vi "Log_Calib_Points.vi"(3 "Instrument type":T1=enum."Cross wire velocity", 4 "Root name":string, 5 "Calib file":path=path "/iMac_3 HD/Users/Hong(6%)/calib/XW Ch 1 7_10_02_6") -> ()   [LabVIEW 2010]
uses:
  Controls/Cal_Inst_type.ctl
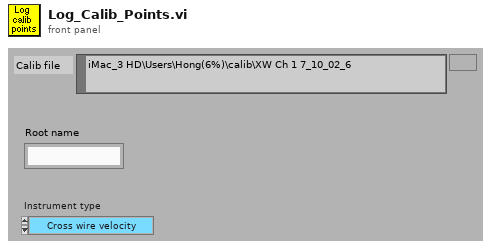
[diagram p1: front panel]
types:
  T1 = typedef "Cal_Inst_type.ctl" = enum16{"Propeller anemometer", "Pressure Transducer", "Hot wire", "Cross wire velocity", "Cross wire angle", "Generic Linear", "Generic Polynomial", "Generic BackPoly", "Fast FID", "Thermocouple", "Cold wire", "Pulsed Wire"}
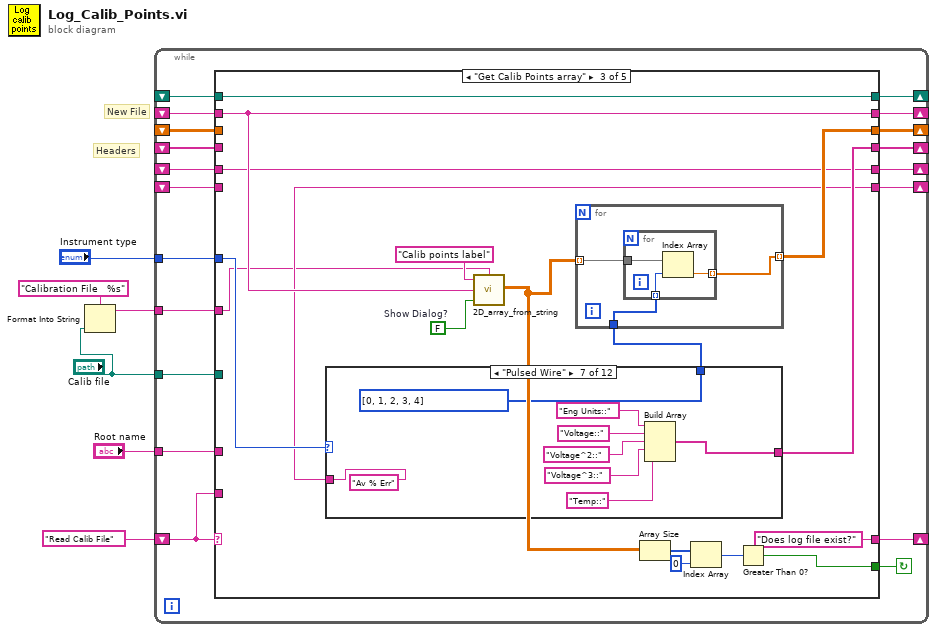
[diagram p0: block diagram]
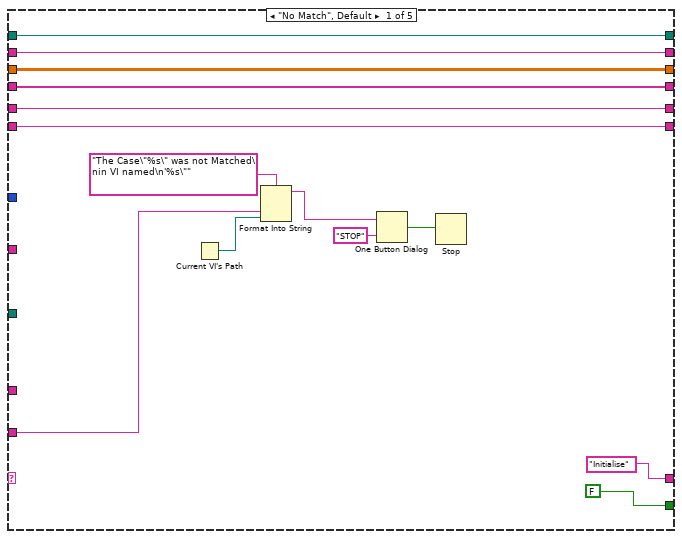
[diagram p2: hidden frame]
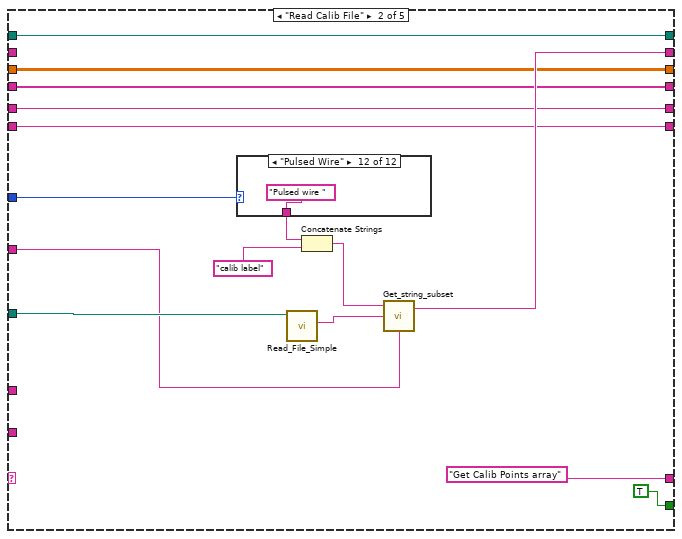
[diagram p3: hidden frame]
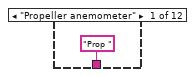
[diagram p4: hidden frame]
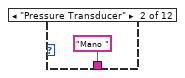
[diagram p5: hidden frame]
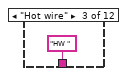
[diagram p6: hidden frame]
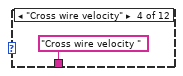
[diagram p7: hidden frame]
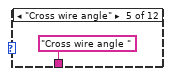
[diagram p8: hidden frame]
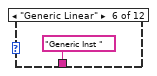
[diagram p9: hidden frame]
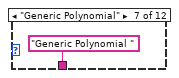
[diagram p10: hidden frame]
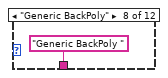
[diagram p11: hidden frame]
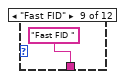
[diagram p12: hidden frame]
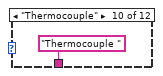
[diagram p13: hidden frame]
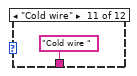
[diagram p14: hidden frame]
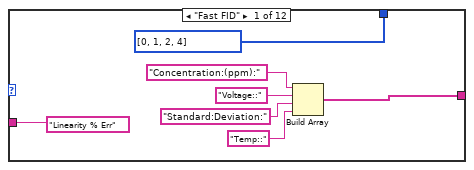
[diagram p15: hidden frame]
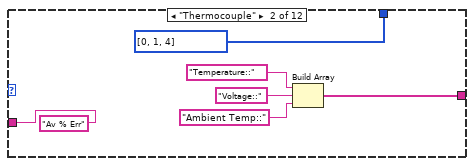
[diagram p16: hidden frame]
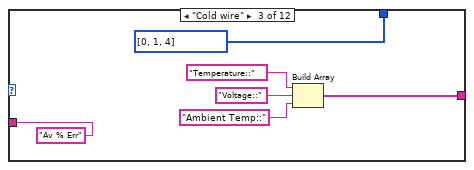
[diagram p17: hidden frame]
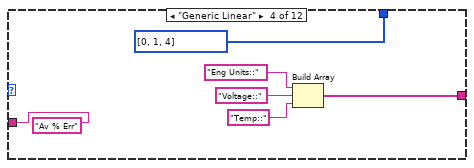
[diagram p18: hidden frame]
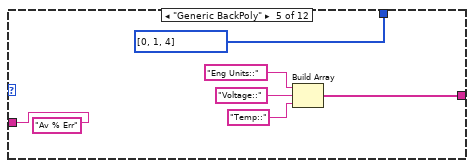
[diagram p19: hidden frame]
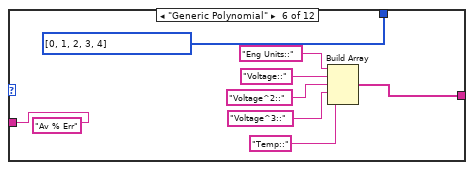
[diagram p20: hidden frame]
diagram:
  # "New File"
  # "Headers"
  n1 = Format Into String(format string="Calibration File   %s", "Calib file") -> (resulting string=w1:string)  [unwired: 2 in, 1 out]
  n2 = while {
    tunnel: "Calib file" -> [w15]
    shift-left: _ -> [w16]
    shift-right: [w17] -> _
    shift-left: _ -> [w18]
    shift-right: [w20] -> _
    tunnel: "Instrument type" -> [w22]
    shift-left: _ -> [w19]
    shift-right: [w21] -> _
    shift-left: "Read Calib File" -> [w23]
    shift-right: [w24] -> _
    tunnel: "Root name" -> [w14]
    shift-right: [w13] -> _
    shift-left: _ -> [w12]
    shift-right: [w11] -> _
    shift-left: _ -> [w10]
    shift-right: [w9] -> _
    shift-left: _ -> [w8]
    tunnel: w1 -> [w7]
    stop <- w25 continue-if-true
    n3 = case shown="\"Get Calib Points array\"" w23 {
      tunnel: [FALSE TRUE w77 TRUE FALSE] -> w25
      tunnel: ["Initialise" "Get Calib Points array" "Does log file exist?" "Append to log file" "End"] -> w24
      tunnel: w23 -> [w34 _ _ _ _]
      tunnel: w22 -> [_ w50 w81 _ _]
      tunnel: [w31 w49 w76 w176 w207] -> w21
      tunnel: [w30 w44 w70 w179 w220] -> w20
      tunnel: w19 -> [w31 _ w76 w176 w207]
      tunnel: w18 -> [w30 w44 _ w179 w220]
      tunnel: [w29 w48 w73 w180 w217] -> w17
      tunnel: w16 -> [w29 w48 _ w180 w217]
      tunnel: w15 -> [_ w41 _ _ w216]
      tunnel: w14 -> [_ _ _ w172 _]
      tunnel: [w28 w45 w71 w170 w199] -> w13
      tunnel: w12 -> [w28 w45 w71 _ w199]
      tunnel: [w27 w43 w69 w177 w214] -> w11
      tunnel: w10 -> [w27 w43 w69 _ w214]
      tunnel: [w26 w42 w68 w175 w200] -> w9
      tunnel: w8 -> [w26 w42 _ w175 w200]
      tunnel: w7 -> [_ w40 w67 _ _]
      frame "No Match", Default {
        n4 = Current VI's Path() -> (path=w33:path)
        n5 = Format Into String(format string="The Case\"%s\" was not Matched\nin VI named\n'%s\"" ("Format String"), w34, w33) -> (resulting string=w37:string)  [unwired: 2 in, 1 out]
        n6 = One Button Dialog(message=w37, button name ("OK")="STOP") -> (true=w35:bool)
        n7 = Stop(stop? (T)=w35) -> ()
      }
      frame "Read Calib File" {
        n8 = case shown="\"Pulsed Wire\"" w50 {
          tunnel: ["Prop " "Mano " "HW " "Cross wire velocity " "Cross wire angle " "Generic Inst " "Generic Polynomial " "Generic BackPoly " "Fast FID " "Thermocouple " "Cold wire " "Pulsed wire "] -> w51
          frame "Propeller anemometer" {
          }
          frame "Pressure Transducer" {
          }
          frame "Hot wire" {
          }
          frame "Cross wire velocity" {
          }
          frame "Cross wire angle" {
          }
          frame "Generic Linear" {
          }
          frame "Generic Polynomial" {
          }
          frame "Generic BackPoly" {
          }
          frame "Fast FID" {
          }
          frame "Thermocouple" {
          }
          frame "Cold wire" {
          }
          frame "Pulsed Wire" {
          }
        }
        n9 = call "Read_File_Simple.vi"("Filename"=w41) -> ("string"=w53:string)  [unwired: 2 in, 7 out]
        n10 = Concatenate Strings(w51, "calib label") -> (w47:string)
        n11 = call "Get_string_subset.vi"("String Name"=w40, "String to split"=w53, "File Label"=w47) -> ("Output string"=w49:string)  [unwired: 1 in, 1 out]
      }
      frame "Get Calib Points array" {
        w83 = FALSE  # Show Dialog?
        n12 = case shown="\"Pulsed Wire\"" w81 {
          tunnel: [i32[] [0, 1, 2, 4] i32[] [0, 1, 4] i32[] [0, 1, 4] i32[] [0, 1, 4] i32[] [0, 1, 4] i32[] [0, 1, 2, 3, 4] i32[] [0, 1, 2, 3, 4] i32[] [0, 1, 2, 3, 4] i32[] [0, 1, 2, 4] i32[] [0, 1, 4] i32[] [0, 1, 4] i32[] [0, 1, 4]] -> w75
          tunnel: [w93 w98 w104 w110 w116 w125 w133 w141 w148 w154 w160 w166] -> w70
          tunnel: ["Linearity % Err" "Av % Err" "Av % Err" "Av % Err" "Av % Err" "Av % Err" "Av % Err" "Av % Err" "Av % Err" "Av % Err" "Av % Err" "Av % Err"] -> w68
          frame "Fast FID" {
            n13 = Build Array("Concentration:(ppm):" ("Substring"), "Voltage::" ("Substring"), "Standard:Deviation:" ("Substring"), "Temp::" ("Substring")) -> (w93:string[])
          }
          frame "Thermocouple" {
            n14 = Build Array("Temperature::" ("Substring"), "Voltage::" ("Substring"), "Ambient Temp::" ("Substring")) -> (w98:string[])
          }
          frame "Cold wire" {
            n15 = Build Array("Temperature::" ("Substring"), "Voltage::" ("Substring"), "Ambient Temp::" ("Substring")) -> (w104:string[])
          }
          frame "Generic Linear" {
            n16 = Build Array("Eng Units::" ("Substring"), "Voltage::" ("Substring"), "Temp::" ("Substring")) -> (w110:string[])
          }
          frame "Generic BackPoly" {
            n17 = Build Array("Eng Units::" ("Substring"), "Voltage::" ("Substring"), "Temp::" ("Substring")) -> (w116:string[])
          }
          frame "Generic Polynomial" {
            n18 = Build Array("Eng Units::" ("Substring"), "Voltage::" ("Substring"), "Voltage^2::" ("Substring"), "Voltage^3::" ("Substring"), "Temp::" ("Substring")) -> (w125:string[])
          }
          frame "Pulsed Wire" {
            n19 = Build Array("Eng Units::" ("Substring"), "Voltage::" ("Substring"), "Voltage^2::" ("Substring"), "Voltage^3::" ("Substring"), "Temp::" ("Substring")) -> (w133:string[])
          }
          frame "Cross wire angle" {
            n20 = Build Array("Angle:(degrees):" ("Substring"), "HW1 Voltage::" ("Substring"), "HW2 Voltage::" ("Substring"), "Ref velocity", "Temp::" ("Substring")) -> (w141:string[])
          }
          frame "Cross wire velocity" {
            n21 = Build Array("Velocity::" ("Substring"), "HW1 Voltage::" ("Substring"), "HW2 Voltage::" ("Substring"), "Temp::" ("Substring")) -> (w148:string[])
          }
          frame "Hot wire" {
            n22 = Build Array("Velocity::" ("Substring"), "HW Voltage::" ("Substring"), "Temp::" ("Substring")) -> (w154:string[])
          }
          frame "Propeller anemometer" {
            n23 = Build Array("Velocity::" ("Substring"), "Voltage::" ("Substring"), "Temp::" ("Substring")) -> (w160:string[])
          }
          frame "Pressure Transducer" {
            n24 = Build Array("Pressure::" ("Substring"), "Voltage::" ("Substring"), "Temp::" ("Substring")) -> (w166:string[])
          }
        }
        n25 = call "2D_array_from_string.vi"("String Name"=w67, "Show Dialog?"=w83, "Input string"=w76, "Array title"="Calib points label") -> ("2D data array"=w74:dbl[][])
        n26 = for {
          tunnel: w75 -> [w86]
          tunnel: w74 -> [w85] mode=indexing
          tunnel: [w84] -> w73 mode=indexing
          n27 = for {
            tunnel: w86 -> [w89] mode=indexing
            tunnel: w85 -> [w88]
            tunnel: [w87] -> w84 mode=indexing
            n28 = Index Array(array=w88, index=w89) -> (element=w87:dbl)
          }
        }
        n29 = Array Size(array=w74) -> (size(s)=w80:i32[])
        n30 = Index Array(array=w80, index=0 ("Index")) -> (element=w78:i32)
        n31 = Greater Than 0?(x=w78) -> (x > 0?=w77:bool)
      }
      frame "Does log file exist?" {
        n32 = call "Remove_underscores_at_ends.vi"("String in"=w172) -> ("String out"=w173:string)
        n33 = call "Create_Error_log_folders.vi"("Log Folder"="Calib_Points", "Log Filename"=w173) -> ("Server copy Location"=w170:path)  [unwired: 1 in, 2 out]
        n34 = call "Does_file_exist_(simple).vi"("Pathname"=w170) -> ("exists?"=w171:bool)
        n35 = case shown="False" w171 {
          tunnel: w179 -> [w192 _]
          tunnel: [w193 ""] -> w177
          tunnel: w175 -> [w186 _]
          frame False {
            n36 = Concatenate Strings(w186, "::" ("string")) -> (w184:string)
            n37 = Build Array (concatenate)("Date::" ("Substring"), "Time::" ("Substring"), "Seconds:Since:1904" ("Substring"), "Calib:filename:" ("Substring"), w192, w184, "Drift:%:", "Drift:Interval:Minutes") -> (w191:string[])
            n38 = call "Ch_names_to_rows.vi"("Channel Names"=w191) -> ("3 Row names"=w194:string[][])
            n39 = Array To Spreadsheet String(array=w194, 3:"%s" ("format string")) -> (spreadsheet string=w193:string)  [unwired: 1 out]
          }
          frame True {
          }
        }
        n40 = call "Remember_Results_Files.vi"("Filename to Remember"=w170) -> ()  [unwired: 1 out]
      }
      frame "Append to log file" {
        w197 = TRUE  # append to file? (new file:F)
        n41 = call "Get_Characters_from_string.vi"("Input string"=w207, "Variable name"=w200) -> ("Value"=w206:string)  [unwired: 1 in, 1 out]
        n42 = Strip Path(path=w216) -> (name=w203:string)  [unwired: 1 out]
        n43 = Concatenate Strings(w203, "_Drift_Place_Holder" ("Substring")) -> (w202:string)
        n44 = call "Get_Characters_from_string.vi"("Input string"=w207, "Variable name"="Time") -> ("Value"=w209:string)  [unwired: 1 in, 1 out]
        n45 = call "Get_Characters_from_string.vi"("Input string"=w207, "Variable name"="Seconds since 1/1/04") -> ("Value"=w208:string)  [unwired: 1 in, 1 out]
        n46 = call "Get_Characters_from_string.vi"("Input string"=w207, "Variable name"="Date") -> ("Value"=w210:string)  [unwired: 1 in, 1 out]
        n47 = Concatenate Strings(w203, "_Interval_Place_Holder" ("Substring")) -> (w201:string)
        n48 = for {
          tunnel: w217 -> [w232] mode=indexing
          tunnel: w203 -> [w226]
          tunnel: [w230] -> w215 mode=indexing
          tunnel: w210 -> [w229]
          tunnel: w209 -> [w228]
          tunnel: w208 -> [w227]
          tunnel: w206 -> [w225]
          tunnel: w202 -> [w224]
          tunnel: w201 -> [w223]
          n49 = Number To Exponential String(number=w232, precision (6)=i16 10) -> (E-format string=w231:string[])  [unwired: 2 out]
          n50 = Build Array (concatenate)(w229, w228, w227, w226, w231, w225, w224, w223) -> (w230:string[])
        }
        n51 = Array To Spreadsheet String(array=w215, 3:"%s" ("format string")) -> (spreadsheet string=w221:string)  [unwired: 1 out]
        n52 = Concatenate Strings(w214, w221) -> (w198:string)
        n53 = call "Write_File_Simple.vi"("append to file? (new file:F)"=w197, "character string"=w198, "file path"=w199) -> ()  [unwired: 2 out]
      }
    }
  }
